vi "Fail If Specific Error.vi"(6 "Error Codes":i32[](array[numeric]), 7 "Description":string, 8 "error in (no error)":errorcluster, 10 "Assert error":errorcluster, 11 "LUnit Test Case In":refnum<class "LUnit Test Case.lvclass">) -> (0 "error out":errorcluster, 3 "LUnit Test Case Out":refnum<class "LUnit Test Case.lvclass">)   [LabVIEW 2020, in "Advanced Assertions.lvlib"]
doc: "Generates a fail result for the calling test method if the inputs contains an error with status \"True\". Using the Error Codes input it is possible to select which specific error codes to test for. A description may be provided to the result."
uses:
  Advanced Assertions.lvlib
  LUnit Test Case.lvclass
  LUnit Test Case.lvclass/LUnit Test Case.ctl
  c764aba1-6191-4a45-99b6-9f14aa7c11f7.vi
  Core/LUnit Test Case/Private/Append Pass Result.vi
  Core/LUnit Test Case/Private/Append Fail Result.vi
  Core/LUnit Test Case/Private/Run In UI.vi
  <vilib>/Utility/error.llb/Clear Errors.vi
  <vilib>/Comparison/Equal/Equal Functor/Equal Functor.lvclass
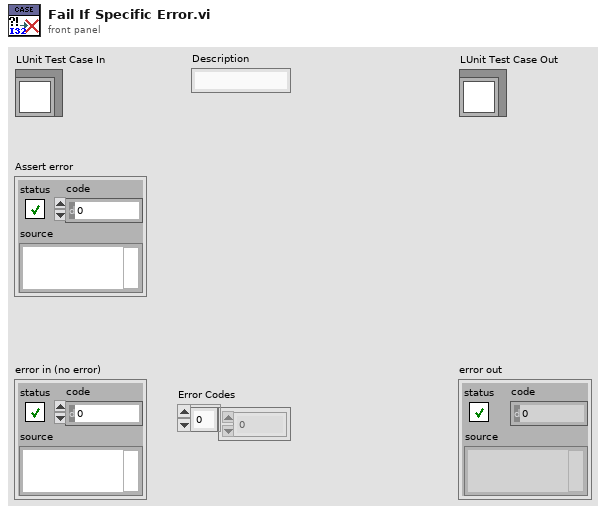
[diagram p1: front panel]
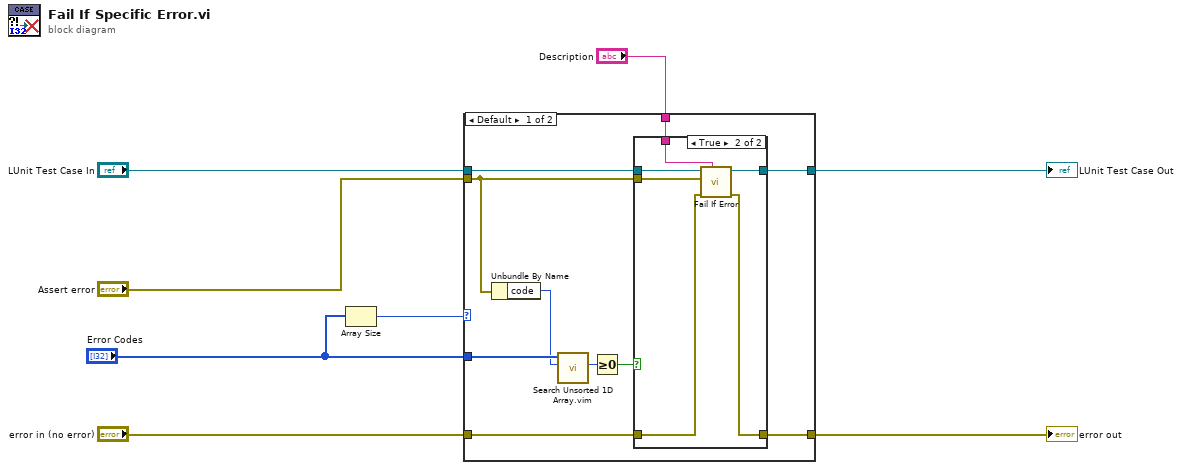
[diagram p0: block diagram]
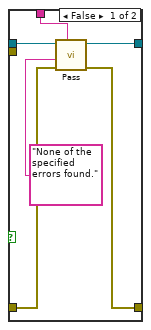
[diagram p2: hidden frame]
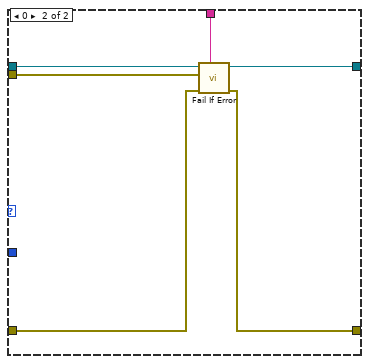
[diagram p3: hidden frame]
diagram:
  n1 = Array Size(array="Error Codes") -> (size(s)=w1:i32)
  n2 = case shown="Default" w1 {
    tunnel: "LUnit Test Case In" -> [w18 w36]
    tunnel: [w15 w35] -> w6
    tunnel: [w16 w34] -> w5
    tunnel: "error in (no error)" -> [w17 w33]
    tunnel: "Assert error" -> [w10 w32]
    tunnel: "Description" -> [w14 w31]
    tunnel: "Error Codes" -> [w13 _]
    frame Default {
      n3 = Unbundle By Name(w10) -> ("code"=w9:i32)
      n4 = call "Search Unsorted 1D Array.vim"("element"=w9, "unsorted 1D array"=w13) -> ("index of element"=w12:i32)  [unwired: 9 in]
      n5 = Greater Or Equal To 0?(x=w12) -> (x >= 0?=w11:bool)
      n6 = case shown="True" w11 {
        tunnel: w18 -> [w21 w30]
        tunnel: w10 -> [_ w29]
        tunnel: w17 -> [w24 w28]
        tunnel: [w23 w27] -> w16
        tunnel: [w22 w26] -> w15
        tunnel: w14 -> [w20 w25]
        frame False {
          n7 = call "Pass.vi"("Description"=w20, "error in (no error)"=w24, "Message"="None of the specified errors found.", "LUnit Test Case In"=w21) -> ("error out"=w23:errorcluster, "LUnit Test Case Out"=w22:refnum<class "LUnit Test Case.lvclass">)  [unwired: 6 in]
        }
        frame True {
          n8 = call "Fail If Error.vi"("Description"=w25, "error in (no error)"=w28, "Assert error"=w29, "LUnit Test Case In"=w30) -> ("error out"=w27:errorcluster, "LUnit Test Case Out"=w26:refnum<class "LUnit Test Case.lvclass">)  [unwired: 6 in]
        }
      }
    }
    frame 0 {
      n9 = call "Fail If Error.vi"("Description"=w31, "error in (no error)"=w33, "Assert error"=w32, "LUnit Test Case In"=w36) -> ("error out"=w34:errorcluster, "LUnit Test Case Out"=w35:refnum<class "LUnit Test Case.lvclass">)  [unwired: 6 in]
    }
  }
  "error out" <- w5
  "LUnit Test Case Out" <- w6
